vi "Datei speichern auf cRio.vi"(4 "Password":string="iag", 6 "User Name":string="iag", 7 "IP Adresse":string, 8 "error in":errorcluster, 9 "Dateien":string[](array[string]), 10 "Pfad PLC":string, 11 "Ordnerpfad PC":path) -> (0 "error out":errorcluster, 1 "Dateipfad PC":path[](array[path]), 3 "ohne Fehler":bool)   [LabVIEW 2020, in "FTP WebDAV.lvlib"]
doc: "Speichert ein Array von Dateinamen vom PC auf die cRIO.\nftp ode webDAV (je nach FGV FTP WebDAV.vi Ausgang).\n\nSowohl für webDAV als auch ftp genügt diese URL/Pfad Notation:\nhome/lvuser/natinst/bin/ oder c/KonfigIAG/\n(vorne kein / notwendig, hinten schon ! - ftp ist das egal, bei webDAV wird http://IP/files/ intern voran gestellt)\n\nriw - 2019-02-22"
uses:
  FTP WebDAV.lvlib
  Aktionen FTP WebDAV.ctl
  <vilib>/WebDAVClient/Simple Put File.vi
  <vilib>/FTP/NI_FTP.lvlib
  <vilib>/WebDAVClient/NI_WebDAV.lvlib
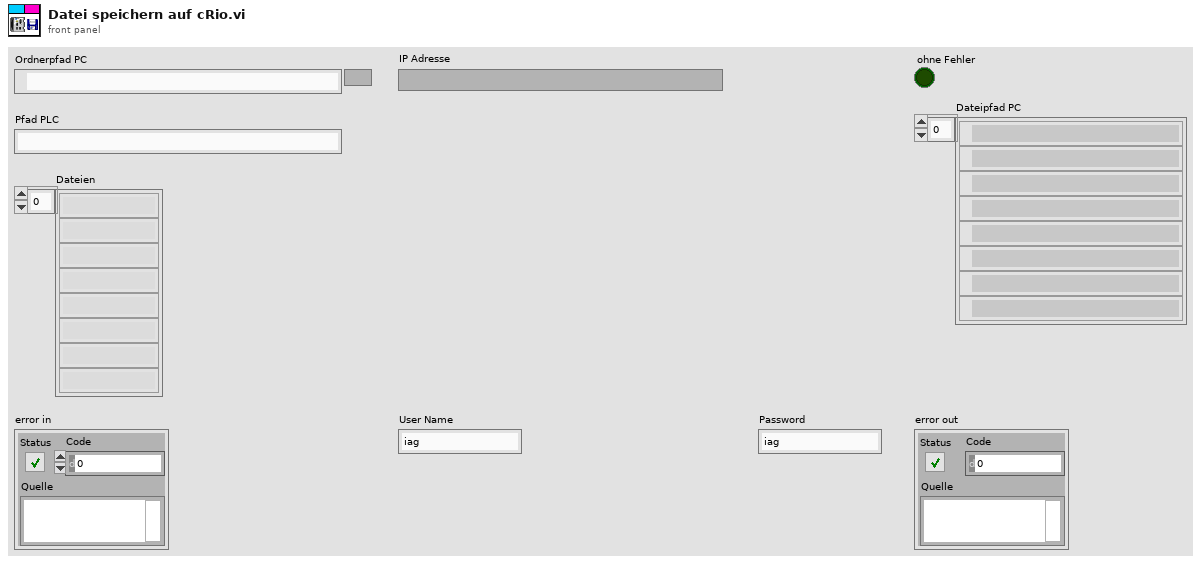
[diagram p1: front panel]
types:
  T1 = typedef "FTP WebDAV.lvlib/Aktionen FTP WebDAV.ctl" = enum16{"lesen", "erkennen"}
  T2 = typedef "FTP WebDAV.lvlib/Enum FTP WebDAV.ctl" = enum16{" nix", "ftp", "webDAV"}
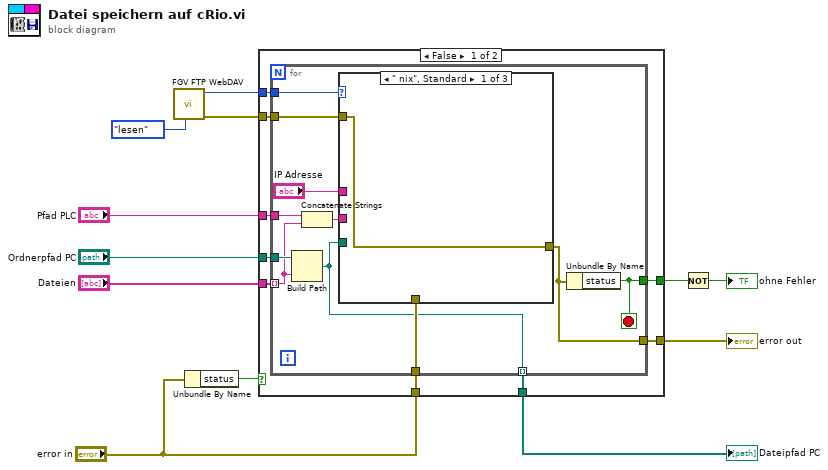
[diagram p0: block diagram]
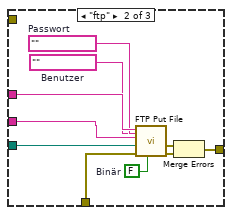
[diagram p2: hidden frame]
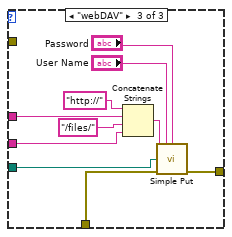
[diagram p3: hidden frame]
diagram:
  n1 = call "FGV FTP WebDAV.vi"("Aktionen"=Aktionen_FTP_WebDAV."lesen") -> ("Fehler (Ausgang)"=w2:errorcluster, "ftp webDAV"=w1:T2)  [unwired: 6 in, 3 out]
  n2 = Unbundle By Name("error in") -> ("status"=w8:bool)
  n3 = case shown="False" w8 {
    selector: w8 -> [_ w54]
    tunnel: "Ordnerpfad PC" -> [w21 _]
    tunnel: "Pfad PLC" -> [w20 _]
    tunnel: "Dateien" -> [w19 _]
    tunnel: [w18 w54] -> w6
    tunnel: [w17 w55] -> w4
    tunnel: "error in" -> [w16 w55]
    tunnel: [w15 _] -> w9
    tunnel: w1 -> [w14 _]
    tunnel: w2 -> [w13 _]
    frame False {
      n4 = for {
        tunnel: w21 -> [w32]
        tunnel: w20 -> [w23]
        tunnel: w19 -> [w24] mode=indexing
        tunnel: [w28] -> w18
        tunnel: [w31] -> w17
        tunnel: w16 -> [w30]
        tunnel: [w29] -> w15 mode=indexing
        tunnel: w14 -> [w26]
        tunnel: w13 -> [w25]
        stop <- w28 stop-if-true
        n5 = Build Path(base path=w32, name or relative path=w24) -> (appended path=w29:path)
        n6 = Concatenate Strings(w23, w24) -> (w22:string)
        n7 = case shown="\" nix\", Standard" w26 {
          tunnel: [w33 w43 w53] -> w31
          tunnel: w30 -> [_ w42 w52]
          tunnel: w29 -> [_ w41 w51]
          tunnel: "IP Adresse" -> [_ w40 w50]
          tunnel: w22 -> [_ w34 w44]
          tunnel: w25 -> [w33 _ _]
          frame " nix", Default {
          }
          frame "ftp" {
            w37 = ""  # Passwort
            w36 = ""  # Benutzer
            w35 = FALSE  # Binär
            n8 = call <vilib>:"FTP Put File.vi"("password"=w37, "binary (F)"=w35, "user"=w36, "error in (no error)"=w42, "local path"=w41, "remote path"=w34, "host"=w40) -> ("error out"=w38:errorcluster, "file error"=w39:errorcluster)  [unwired: 3 in]
            n9 = Merge Errors(w39, w38) -> (w43:errorcluster)
          }
          frame "webDAV" {
            n10 = Concatenate Strings("http://" ("String"), w50, "/files/" ("String"), w44) -> (w47:string)
            n11 = call-poly <vilib>:"Simple Put.vi"("file uri"=w47, "username"="User Name", "password"="Password", "local file path"=w51, "error in (no error)"=w52) -> ("error out"=w53:errorcluster)  [unwired: 9 in, 1 out]
          }
        }
        n12 = Unbundle By Name(w31) -> ("status"=w28:bool)
      }
    }
    frame True {
    }
  }
  "error out" <- w4
  "Dateipfad PC" <- w9
  n13 = Not(x=w6) -> (.not. x?=→"ohne Fehler":bool)
